vi "Queue Transport.vi"(6 "Refs":refnum<class "Refs.lvclass">, 7 "Actor in":refnum<class "Actor.lvclass">, 9 "Actor Ref":refnum<vi>, 10 "Spawn":refnum<class "Spawn.lvclass">) -> (0 "Error out":errorcluster, 5 "Actor out":refnum<class "Actor.lvclass">)   [LabVIEW 2025, in "jettl.lvlib" / "Transport.lvlib" / "Queue.lvlib"]
uses:
  Queue.lvlib
  Spawn/Spawn/Spawn.lvclass
  Actor/Actor.lvclass
  Refs/Refs.lvclass
  jettl.lvlib
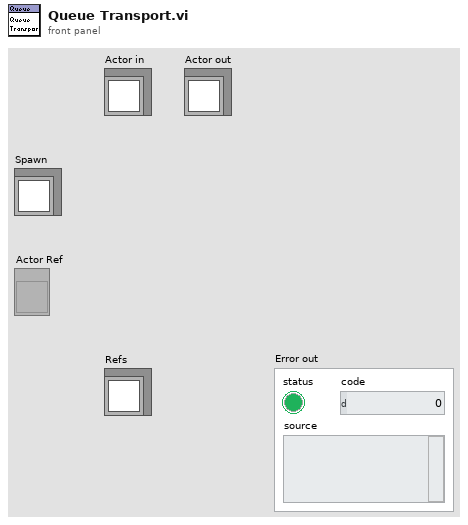
[diagram p1: front panel]
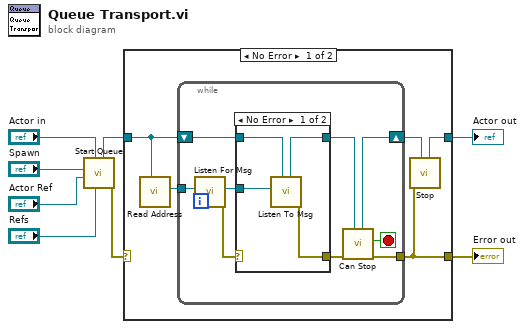
[diagram p0: block diagram]
diagram:
  n1 = call "Start Queue.vi"("Refs"="Refs", "Actor in"="Actor in", "Actor Ref"="Actor Ref", "Spawn"="Spawn") -> ("Error out"=w4:errorcluster, "Actor out"=w5:refnum<class "Actor.lvclass">)  [unwired: 6 in]
  n2 = case shown="No Error" w4 {
    selector: w4 -> [_ w29]
    tunnel: [w11 w30] -> w7
    tunnel: w5 -> [w10 w30]
    tunnel: [w13 w29] -> w8
    frame No Error {
      n3 = call "Read Address.vi"("Actor"=w10) -> ("Address"=w9:refnum<data-value>)  [unwired: 10 in]
      n4 = while {
        shift-right: [w20] -> w12
        shift-left: w10 -> [w18]
        tunnel: [w21] -> w13
        tunnel: w9 -> [w16]
        stop <- w19 stop-if-true
        n5 = call "Listen For Msg.vi"("Address"=w16) -> ("Error out"=w14:errorcluster, "Msg"=w15:refnum<class "Msg.lvclass">)  [unwired: 9 in]
        n6 = case shown="No Error" w14 {
          selector: w14 -> [_ w27]
          tunnel: [w23 w27] -> w22
          tunnel: w18 -> [w26 w28]
          tunnel: [w24 w28] -> w17
          tunnel: w15 -> [w25 _]
          frame No Error {
            n7 = call "Listen To Msg.vi"("Actor in"=w26, "Msg"=w25) -> ("Error out"=w23:errorcluster, "Actor out"=w24:refnum<class "Actor.lvclass">)  [unwired: 7 in, 1 out]
          }
          frame Error {
          }
        }
        n8 = call "Can Stop.vi"("Actor in"=w17, "Error in"=w22) -> ("Error out"=w21:errorcluster, "Stop"=w19:bool, "Actor out"=w20:refnum<class "Actor.lvclass">)  [unwired: 7 in]
      }
      n9 = call "Stop.vi"("Actor in"=w12, "Error in"=w13) -> ("Actor out"=w11:refnum<class "Actor.lvclass">)  [unwired: 9 in]
    }
    frame Error {
    }
  }
  "Error out" <- w8
  "Actor out" <- w7
